vi "Initialize Custom Device.vi"(8 "error in":errorcluster, 11 "custom device ref":T1=18446744073709551615 format="%.0x") -> (0 "error out":errorcluster, 3 "custom device ref out":T1 format="%.0x")   [LabVIEW 2020, in "AIM ARINC 664 Scripting.lvlib"]
uses:
  AIM ARINC 664 Scripting.lvlib
  <vilib>/NI VeriStand/Custom Device API/Custom Device Item Ref.ctl
  <vilib>/NI VeriStand/Custom Device API/Custom Device API.lvlib
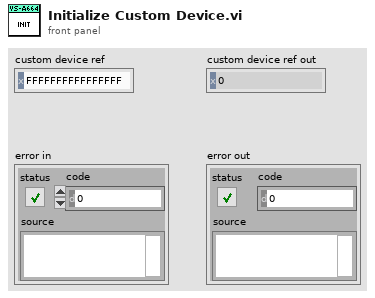
[diagram p1: front panel]
types:
  T1 = typedef "Custom Device API.lvlib/Custom Device Item Ref.ctl" = u64
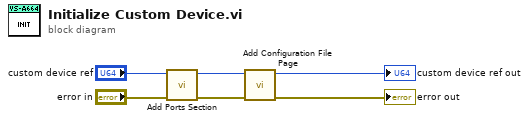
[diagram p0: block diagram]
diagram:
  n1 = call "Add Ports Section.vi"("error in"="error in", "custom device Ref"="custom device ref") -> ("error out"=w5:errorcluster, "custom device Ref out"=w3:T1)  [unwired: 8 in]
  n2 = call "Add Configuration File Page.vi"("error in"=w5, "custom device ref in"=w3) -> ("error out"=→"error out":errorcluster, "custom device ref out"=→"custom device ref out":T1)  [unwired: 8 in]
